vi "Build SwarmOutputArray.vi"(8 "AllTagDistancesArray":T2(array[cluster]), 10 "Solution Vector":dbl[](array[numeric])=[77.46091556296253, 28.48740055495817, 55.01909042958664, 38.62900138602302, 48.65901937283867, -41.404820463734396]) -> (1 "SwarmOutputArray":T1(array[cluster])=[{"TagIDFrom"=0.0, "EstimatedX"=77.46091556296253, "EstimatedY"=28.48740055495817, "TagIDDistanceClusterArray"=[{"TagIDTo"=1.0, "Distance"=4.082563465494822}, {"TagIDTo"=2.0, "Distance"=7.397690797704779}]}, {"TagIDFrom"=1.0, "EstimatedX"=55.01909042958664, "EstimatedY"=38.62900138602302, "TagIDDistanceClusterArray"=[{"TagIDTo"=2.0, "Distance"=5.764709508348148}]}, {"TagIDFrom"=2.0, "EstimatedX"=48.65901937283867, "EstimatedY"=-41.404820463734396, "TagIDDistanceClusterArray"=[]}])   [LabVIEW 2014]
doc: "Builds the SwarmOutputArray based on the calculations from Estimate All Positions (Swarm)"
uses:
  Tag.lvclass
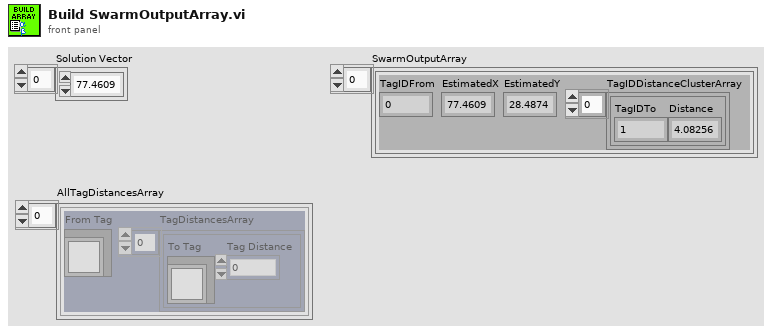
[diagram p1: front panel]
types:
  T1 = cluster{"TagIDFrom":dbl, "EstimatedX":dbl, "EstimatedY":dbl, "TagIDDistanceClusterArray":cluster{"TagIDTo":dbl, "Distance":dbl}[]}[]
  T2 = cluster{"From Tag":refnum<class "Tag.lvclass">, "TagDistancesArray":cluster{"To Tag":refnum<class "Tag.lvclass">, "Tag Distance":dbl}[]}[]
  T3 = cluster{"To Tag":refnum<class "Tag.lvclass">, "Tag Distance":dbl}[]
  T4 = cluster{"Tag ID":dbl, dbl, dbl, "TagIDDistanceClusterArray":cluster{"TagIDTo":dbl, "Distance":dbl}[]}
  T5 = cluster{"Tag ID":dbl, "EstimatedX":dbl, "EstimatedY":dbl, "TagIDDistanceClusterArray":cluster{"TagIDTo":dbl, "Distance":dbl}[]}[]
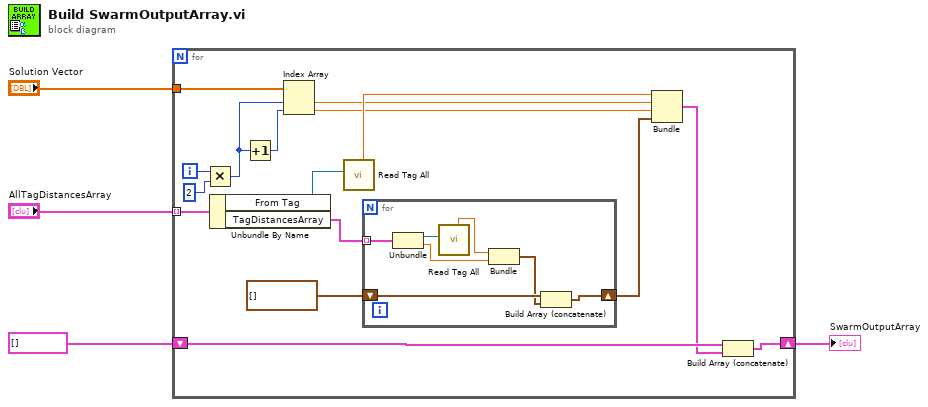
[diagram p0: block diagram]
diagram:
  n1 = for {
    tunnel: "Solution Vector" -> [w20]
    tunnel: "AllTagDistancesArray" -> [w15] mode=indexing
    shift-right: [w9] -> w1
    shift-left: T1 [] ("SwarmOutputArray") -> [w10]
    i -> [w19]
    n2 = Multiply(x=w19, y=2) -> (x*y=w17:i32)
    n3 = Unbundle By Name(w15) -> ("From Tag"=w14:refnum<class "Tag.lvclass">, "TagDistancesArray"=w7:T3)
    n4 = Increment(x=w17) -> (x+1=w16:i32)
    n5 = Index Array(array=w20, index #1=w17, index #2=w16) -> (element #1=w12:dbl, element #2=w11:dbl)
    n6 = call "Read Tag All.vi"("Tag.lvclass"=w14) -> ("Tag ID"=w13:dbl)  [unwired: 5 in, 5 out]
    n7 = for {
      tunnel: w7 -> [w27] mode=indexing
      shift-right: [w24] -> w5
      shift-left: cluster{"TagIDTo":dbl, "Distance":dbl}[] [] ("TagIDDistanceClusterArray") -> [w25]
      n8 = Unbundle(w27) -> ("To Tag"=w26:refnum<class "Tag.lvclass">, "Tag Distance"=w22:dbl)
      n9 = call "Read Tag All.vi"("Tag.lvclass"=w26) -> ("Tag ID"=w23:dbl)  [unwired: 5 in, 5 out]
      n10 = Bundle("Tag ID"=w23, "Tag Distance"=w22) -> (w21:cluster{"Tag ID":dbl, "Tag Distance":dbl})  [unwired: 1 in]
      n11 = Build Array (concatenate)(w25, w21) -> (w24:cluster{"Tag ID":dbl, "Tag Distance":dbl}[])
    }
    n12 = Bundle("Tag ID"=w13, w12, w11, "TagIDDistanceClusterArray"=w5) -> (w8:T4)  [unwired: 1 in]
    n13 = Build Array (concatenate)(w10, w8) -> (w9:T5)
  }
  "SwarmOutputArray" <- w1
